vi "_PC_SaveFile displaySpectrumData.vi"(7 "plotNameArr":string[](array[string]), 8 "error in (no error)":errorcluster, 9 "graphRefnum in":T3, 10 "labelName":T2, 11 "newScanData":T1(array[cluster])) -> (0 "error out":errorcluster, 1 "graphRefnum out":T3)   [LabVIEW 2018]
uses:
  <vilib>/Analysis/baseanly.llb/Mean (DBL).vi
  <vilib>/Analysis/NI_AALBase.lvlib
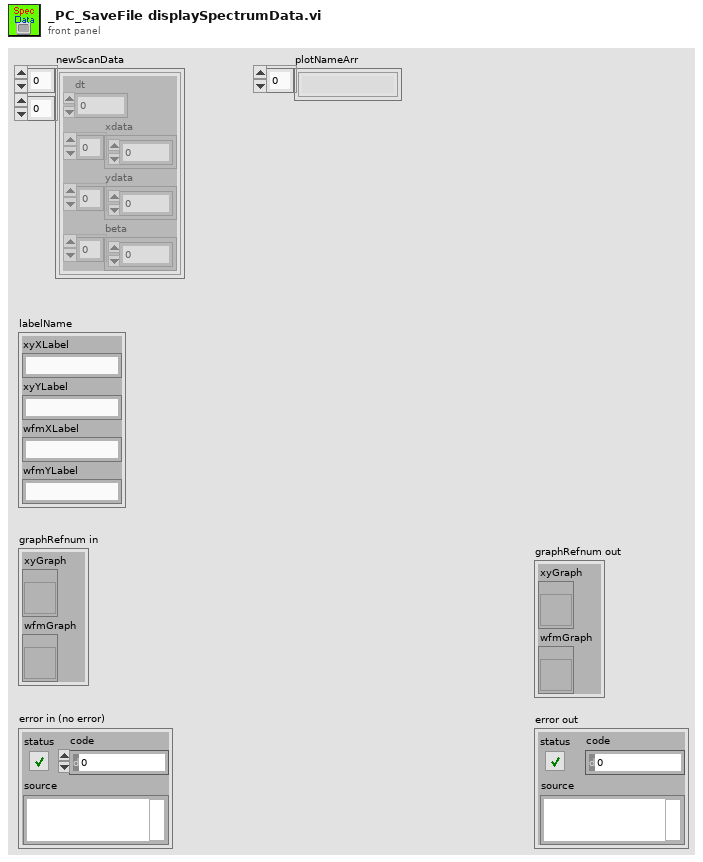
[diagram p1: front panel]
types:
  T1 = cluster{"dt":dbl, "xdata":dbl[], "ydata":sgl[], "beta":dbl[]}[][]
  T2 = cluster{"xyXLabel":string, "xyYLabel":string, "wfmXLabel":string, "wfmYLabel":string}
  T3 = cluster{"xyGraph":refnum<vi>, "wfmGraph":refnum<vi>}
  T4 = cluster{"dt":dbl, "xdata":dbl[], "ydata":sgl[], "beta":dbl[]}[]
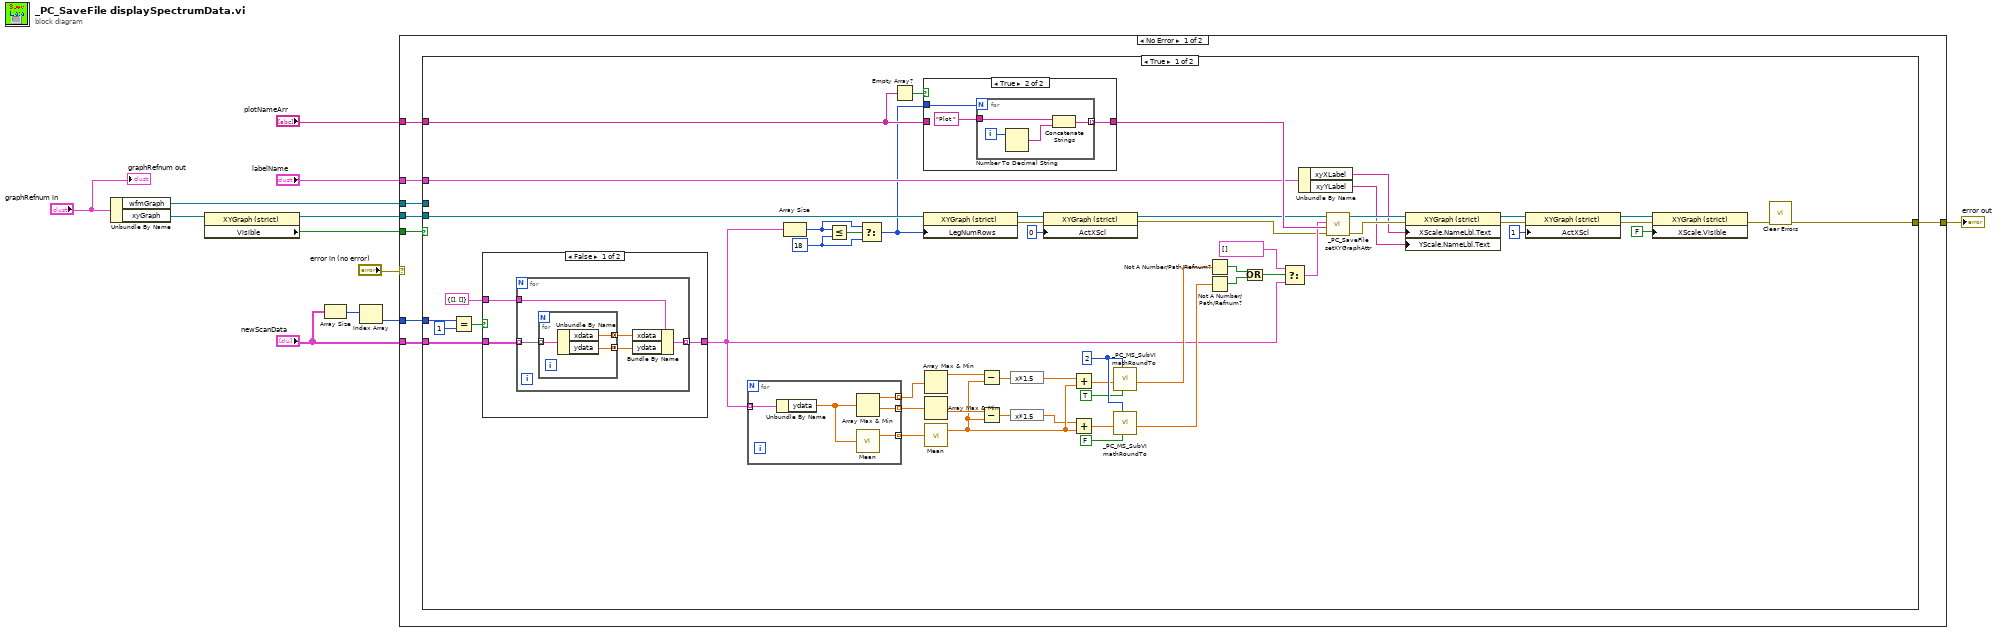
[diagram p0: block diagram]
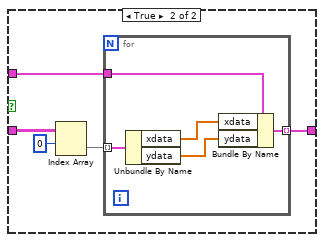
[diagram p2: hidden frame]
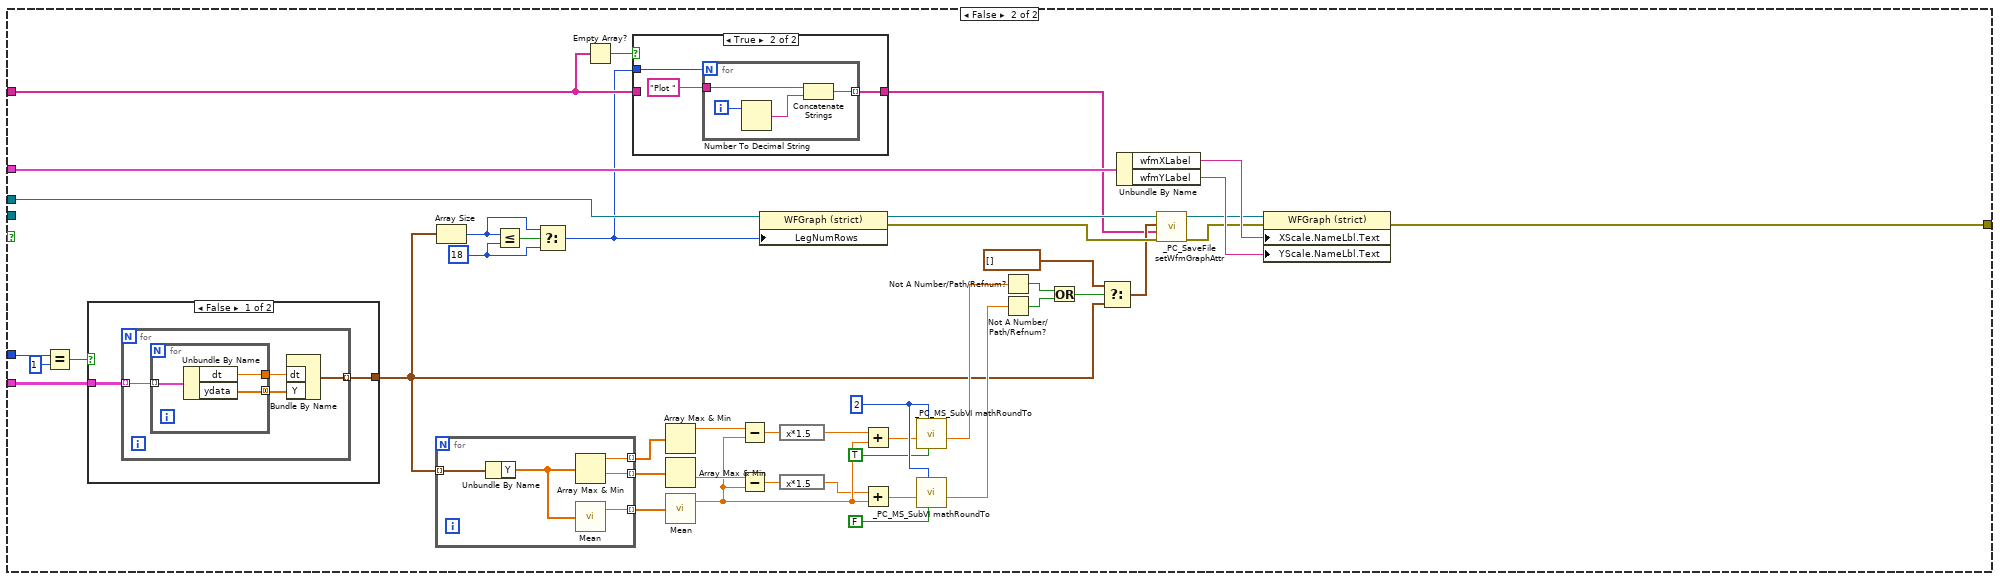
[diagram p4: hidden frame]
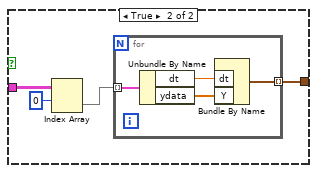
[diagram p5: hidden frame]
diagram:
  n1 = Unbundle By Name("graphRefnum in") -> ("wfmGraph"=w8:refnum<vi>, "xyGraph"=w11:refnum<vi>)
  n2 = property class="XYGraph (strict)"(reference=w11) -> (reference out=w9:refnum<vi>, "Visible"=w10:bool)  [unwired: 1 in, 1 out]
  n3 = Array Size(array="newScanData") -> (size(s)=w2:i32[])
  n4 = Index Array(array=w2) -> (element=w1:i32)  [unwired: 1 in]
  n5 = case shown="No Error" "error in (no error)" {
    selector: "error in (no error)" -> [_ w182]
    tunnel: w10 -> [w18 _]
    tunnel: w9 -> [w20 _]
    tunnel: w8 -> [w16 _]
    tunnel: "labelName" -> [w19 _]
    tunnel: "plotNameArr" -> [w17 _]
    tunnel: [w15 w182] -> w6
    tunnel: "newScanData" -> [w14 _]
    tunnel: w1 -> [w13 _]
    frame No Error {
      n6 = case shown="True" w18 {
        tunnel: w20 -> [w74 _]
        tunnel: w19 -> [w40 w151]
        tunnel: w17 -> [w66 w150]
        tunnel: [w41 w149] -> w15
        tunnel: w16 -> [_ w124]
        tunnel: w14 -> [w26 w111]
        tunnel: w13 -> [w24 w113]
        frame True {
          w28 = 18 ("y")
          w63 = 2 ("Digit")
          n7 = Equal?(x=w24, y=1) -> (x = y?=w22:bool)
          n8 = case shown="False" w22 {
            tunnel: w26 -> [w77 w90]
            tunnel: [w76 w86] -> w25
            tunnel: cluster{"xdata":dbl[], "ydata":sgl[]} {"xdata"=[], "ydata"=[]} -> [w75 w87]
            frame False {
              n9 = for {
                tunnel: w77 -> [w82] mode=indexing
                tunnel: w75 -> [w81]
                tunnel: [w78] -> w76 mode=indexing
                n10 = for {
                  tunnel: w82 -> [w85] mode=indexing
                  tunnel: [w84] -> w80 mode=concatenating
                  tunnel: [w83] -> w79 mode=concatenating
                  n11 = Unbundle By Name(w85) -> ("xdata"=w84:dbl[], "ydata"=w83:sgl[])
                }
                n12 = Bundle By Name(cluster=w81, "xdata"=w80, "ydata"=w79) -> (w78:cluster{"xdata":dbl[], "ydata":sgl[]})
              }
            }
            frame True {
              n13 = Index Array(array=w90, index (row)=0) -> (element=w88:T4)  [unwired: 1 in]
              n14 = for {
                tunnel: w88 -> [w95] mode=indexing
                tunnel: w87 -> [w94]
                tunnel: [w91] -> w86 mode=indexing
                n15 = Unbundle By Name(w95) -> ("xdata"=w93:dbl[], "ydata"=w92:sgl[])
                n16 = Bundle By Name(cluster=w94, "xdata"=w93, "ydata"=w92) -> (w91:cluster{"xdata":dbl[], "ydata":sgl[]})
              }
            }
          }
          n17 = for {
            tunnel: [w100] -> w50 mode=indexing
            tunnel: [w99] -> w51 mode=indexing
            tunnel: w25 -> [w98] mode=indexing
            tunnel: [w97] -> w49 mode=indexing
            n18 = Unbundle By Name(w98) -> ("ydata"=w96:sgl[])
            n19 = Array Max & Min(array=w96) -> (max value=w99:sgl, min value=w100:sgl)  [unwired: 2 out]
            n20 = call-poly <vilib>:"Mean.vi"("X"=w96) -> ("mean"=w97:dbl)  [unwired: 1 out]
          }
          n21 = Array Size(array=w25) -> (size(s)=w29:i32)
          n22 = Less Or Equal?(x=w29, y=w28) -> (x <= y?=w30:bool)
          n23 = Select(t=w29, s=w30, f=w28) -> (s? t:f=w27:i32)
          n24 = Empty Array?(array=w66) -> (empty?=w65:bool)
          n25 = property class="XYGraph (strict)"(reference=w74, "LegNumRows"=w27) -> (reference out=w72:refnum<vi>, error out=w71:errorcluster)  [unwired: 1 in]
          n26 = case shown="True" w65 {
            tunnel: w27 -> [_ w104]
            tunnel: [w101 w102] -> w64
            tunnel: w66 -> [w101 _]
            frame False {
            }
            frame True {
              n27 = for {
                N: w104 -> [_]
                tunnel: "Plot " -> [w106]
                tunnel: [w105] -> w102 mode=indexing
                i -> [w107]
                n28 = Number To Decimal String(number=w107) -> (decimal integer string=w108:string)  [unwired: 1 in]
                n29 = Concatenate Strings(w106, w108) -> (w105:string)
              }
            }
          }
          n30 = Array Max & Min(array=w51) -> (max value=w62:sgl)  [unwired: 3 out]
          n31 = Array Max & Min(array=w50) -> (min value=w61:sgl)  [unwired: 3 out]
          n32 = call-poly <vilib>:"Mean.vi"("X"=w49) -> ("mean"=w58:dbl)  [unwired: 1 out]
          n33 = Subtract(x=w62, y=w58) -> (x-y=w60:dbl)
          n34 = Subtract(x=w61, y=w58) -> (x-y=w59:dbl)
          n35 = expression code="x*1.5"(w60) -> (w56:dbl)
          n36 = expression code="x*1.5"(w59) -> (w57:dbl)
          n37 = property class="XYGraph (strict)"(reference=w72, error in=w71, "ActXScl"=0 ("Active X Scale")) -> (reference out=w32:refnum<vi>, error out=w31:errorcluster)
          n38 = Add(x=w56, y=w58) -> (x+y=w55:dbl)
          n39 = Add(x=w57, y=w58) -> (x+y=w54:dbl)
          n40 = call "_PC_MS_SubVI mathRoundTo.vi"("Up/Down"=TRUE, "Digit"=w63, "Numeric"=w55) -> ("Round to"=w46:dbl)  [unwired: 8 in]
          n41 = call "_PC_MS_SubVI mathRoundTo.vi"("Up/Down"=FALSE, "Digit"=w63, "Numeric"=w54) -> ("Round to"=w45:dbl)  [unwired: 8 in]
          n42 = Not A Number/Path/Refnum?(number/path/refnum=w46) -> (NaN/Path/Refnum?=w48:bool)
          n43 = Not A Number/Path/Refnum?(number/path/refnum=w45) -> (NaN/Path/Refnum?=w47:bool)
          n44 = Or(x=w48, y=w47) -> (x .or. y?=w44:bool)
          n45 = Select(t=cluster{"X":dbl[], "Y":sgl[]}[] [], s=w44, f=w25) -> (s? t:f=w42:cluster{"xdata":dbl[], "ydata":sgl[]}[])
          n46 = Unbundle By Name(w40) -> ("xyXLabel"=w68:string, "xyYLabel"=w67:string)
          n47 = call "_PC_SaveFile setXYGraphAttr.vi"("error in (no error)"=w31, "plot name"=w64, "plot value"=w42, "graph in"=w32) -> ("error out"=w69:errorcluster, "graph out"=w70:refnum<vi>)  [unwired: 6 in]
          n48 = property class="XYGraph (strict)"(reference=w70, error in=w69, "XScale.NameLbl.Text"=w68, "YScale.NameLbl.Text"=w67) -> (reference out=w39:refnum<vi>, error out=w38:errorcluster)
          n49 = property class="XYGraph (strict)"(reference=w39, error in=w38, "ActXScl"=1 ("Active X Scale")) -> (reference out=w36:refnum<vi>, error out=w37:errorcluster)
          n50 = property class="XYGraph (strict)"(reference=w36, error in=w37, "XScale.Visible"=FALSE ("X Scale.Visible")) -> (error out=w33:errorcluster)  [unwired: 1 out]
          n51 = call <vilib>:"Clear Errors.vi"("error in (no error)"=w33) -> ("error out"=w41:errorcluster)  [unwired: 5 in, 1 out]
        }
        frame False {
          w115 = 18 ("y")
          w145 = 2 ("Digit")
          n52 = Equal?(x=w113, y=1) -> (x = y?=w110:bool)
          n53 = case shown="False" w110 {
            tunnel: w111 -> [w153 w164]
            tunnel: [w152 w161] -> w109
            frame False {
              n54 = for {
                tunnel: w153 -> [w157] mode=indexing
                tunnel: [w154] -> w152 mode=indexing
                n55 = for {
                  tunnel: w157 -> [w160] mode=indexing
                  tunnel: [w159] -> w156
                  tunnel: [w158] -> w155 mode=concatenating
                  n56 = Unbundle By Name(w160) -> ("dt"=w159:dbl, "ydata"=w158:sgl[])
                }
                n57 = Bundle By Name("dt"=w156, "Y"=w155) -> (w154:waveform(sgl))  [unwired: 1 in]
              }
            }
            frame True {
              n58 = Index Array(array=w164, index (row)=0) -> (element=w162:T4)  [unwired: 1 in]
              n59 = for {
                tunnel: w162 -> [w168] mode=indexing
                tunnel: [w165] -> w161 mode=indexing
                n60 = Unbundle By Name(w168) -> ("dt"=w167:dbl, "ydata"=w166:sgl[])
                n61 = Bundle By Name("dt"=w167, "Y"=w166) -> (w165:waveform(sgl))  [unwired: 1 in]
              }
            }
          }
          n62 = for {
            tunnel: [w173] -> w132 mode=indexing
            tunnel: [w172] -> w133 mode=indexing
            tunnel: w109 -> [w170] mode=indexing
            tunnel: [w171] -> w131 mode=indexing
            n63 = Unbundle By Name(w170) -> ("Y"=w169:sgl[])
            n64 = Array Max & Min(array=w169) -> (max value=w172:sgl, min value=w173:sgl)  [unwired: 2 out]
            n65 = call-poly <vilib>:"Mean.vi"("X"=w169) -> ("mean"=w171:dbl)  [unwired: 1 out]
          }
          n66 = Array Size(array=w109) -> (size(s)=w116:i32)
          n67 = Less Or Equal?(x=w116, y=w115) -> (x <= y?=w117:bool)
          n68 = Select(t=w116, s=w117, f=w115) -> (s? t:f=w114:i32)
          n69 = Empty Array?(array=w150) -> (empty?=w146:bool)
          n70 = case shown="True" w146 {
            tunnel: w114 -> [_ w177]
            tunnel: [w174 w175] -> w118
            tunnel: w150 -> [w174 _]
            frame False {
            }
            frame True {
              n71 = for {
                N: w177 -> [_]
                tunnel: "Plot " -> [w179]
                tunnel: [w178] -> w175 mode=indexing
                i -> [w180]
                n72 = Number To Decimal String(number=w180) -> (decimal integer string=w181:string)  [unwired: 1 in]
                n73 = Concatenate Strings(w179, w181) -> (w178:string)
              }
            }
          }
          n74 = Array Max & Min(array=w133) -> (max value=w144:sgl)  [unwired: 3 out]
          n75 = Array Max & Min(array=w132) -> (min value=w143:sgl)  [unwired: 3 out]
          n76 = call-poly <vilib>:"Mean.vi"("X"=w131) -> ("mean"=w140:dbl)  [unwired: 1 out]
          n77 = Subtract(x=w144, y=w140) -> (x-y=w142:dbl)
          n78 = Subtract(x=w143, y=w140) -> (x-y=w141:dbl)
          n79 = property class="WFGraph (strict)"(reference=w124, "LegNumRows"=w114) -> (reference out=w123:refnum<vi>, error out=w122:errorcluster)  [unwired: 1 in]
          n80 = expression code="x*1.5"(w142) -> (w138:dbl)
          n81 = expression code="x*1.5"(w141) -> (w139:dbl)
          n82 = Add(x=w138, y=w140) -> (x+y=w137:dbl)
          n83 = Add(x=w139, y=w140) -> (x+y=w136:dbl)
          n84 = call "_PC_MS_SubVI mathRoundTo.vi"("Up/Down"=TRUE, "Digit"=w145, "Numeric"=w137) -> ("Round to"=w128:dbl)  [unwired: 8 in]
          n85 = call "_PC_MS_SubVI mathRoundTo.vi"("Up/Down"=FALSE, "Digit"=w145, "Numeric"=w136) -> ("Round to"=w127:dbl)  [unwired: 8 in]
          n86 = Not A Number/Path/Refnum?(number/path/refnum=w128) -> (NaN/Path/Refnum?=w130:bool)
          n87 = Not A Number/Path/Refnum?(number/path/refnum=w127) -> (NaN/Path/Refnum?=w129:bool)
          n88 = Or(x=w130, y=w129) -> (x .or. y?=w126:bool)
          n89 = Select(t=waveform(sgl)[] [], s=w126, f=w109) -> (s? t:f=w119:waveform(sgl)[])
          n90 = Unbundle By Name(w151) -> ("wfmXLabel"=w148:string, "wfmYLabel"=w147:string)
          n91 = call "_PC_SaveFile setWfmGraphAttr.vi"("error in (no error)"=w122, "plotName"=w118, "plotValue"=w119, "graph in"=w123) -> ("error out"=w121:errorcluster, "graph out"=w120:refnum<vi>)  [unwired: 6 in]
          n92 = property class="WFGraph (strict)"(reference=w120, error in=w121, "XScale.NameLbl.Text"=w148, "YScale.NameLbl.Text"=w147) -> (error out=w149:errorcluster)  [unwired: 1 out]
        }
      }
    }
    frame Error {
    }
  }
  "error out" <- w6
  "graphRefnum out" <- "graphRefnum in"
